vi "rad_Globals.vi"() -> ()   [LabVIEW 2013]
panel:
  in  "RAD File Version":string="5.5.3"
  in  "Release Date":string="August 2014"
  in  "Empty List Message":string="Selected folder is empty."
  in  "RAD Wiki URL":string="http://zone.ni.com/devzone/cda/epd/p/id/5986"
  in  "Msg_NewerVer":string="One or more newer RAD images are present.\nPlease download the latest version of RAD from:"
  in  "Msg_OldVer":string="One or more older RAD images are present.\nPlease convert any older images by selecting \"Convert Images\" from the \"Images\" menu, then specifying either an image file or repository."
  out "ShownImageVersionDialog":bool
  out "Manager Permissions":bool=TRUE
  in  "RAD App Version":string="14.0"
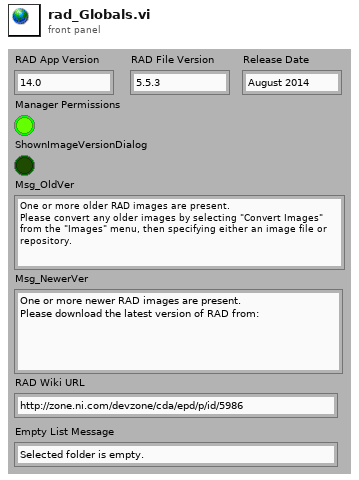
[diagram p1: front panel]
diagram:
